vi "例程25-测量数据的写入.vi"() -> ()   [LabVIEW 2016]
uses:
  <vilib>/measure/NI_MABase.lvlib
panel:
  out "信号":waveform(dbl)(graph)
  in  "Comment":string caption="注释"
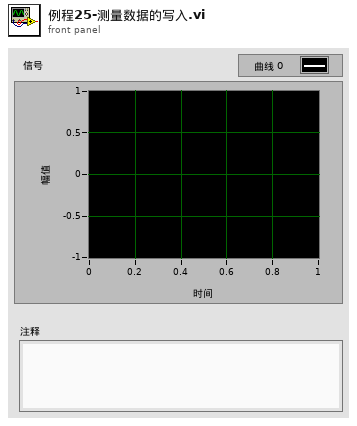
[diagram p1: front panel]
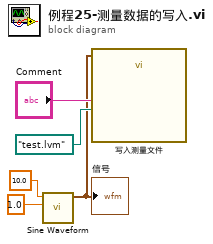
[diagram p0: block diagram]
diagram:
  n1 = call <vilib>:"Sine Waveform.vi"("amplitude"=1.0, "frequency"=10.0) -> ("signal out"=w1:waveform(dbl))  [unwired: 8 in, 1 out]
  "信号" <- w1
  n2 = call "写入测量文件"("Signals"=w1, "Filename"=path "test.lvm", "Comment"="Comment") -> ()  [unwired: 14 in, 3 out]
